vi "poly_lock_fp_updates_lock_vi_ref.vi"(8 "error in":errorcluster, 9 "vi ref":refnum<vi>) -> (0 "error out":errorcluster)   [LabVIEW 2015]
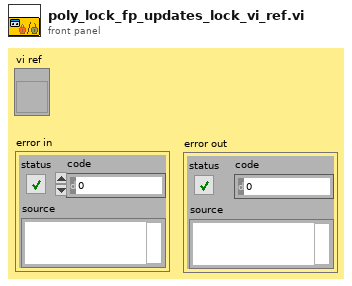
[diagram p1: front panel]
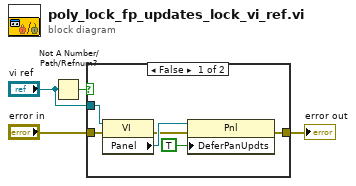
[diagram p0: block diagram]
diagram:
  n1 = Not A Number/Path/Refnum?(number/path/refnum="vi ref") -> (NaN/Path/Refnum?=w1:bool)
  n2 = case shown="False" w1 {
    tunnel: [w9 w11] -> w4
    tunnel: "error in" -> [w7 w11]
    tunnel: "vi ref" -> [w5 _]
    frame False {
      n3 = property class="VI"(reference=w5, error in=w7) -> (error out=w6:errorcluster, "Panel"=w8:refnum<vi>)  [unwired: 1 out]
      n4 = property class="Pnl"(reference=w8, error in=w6, "DeferPanUpdts"=TRUE) -> (error out=w9:errorcluster)  [unwired: 1 out]
    }
    frame True {
    }
  }
  "error out" <- w4
